vi "Write Sleep TS.vi"(8 "error in (no error)":errorcluster, 10 "Sleep":u64, 11 "CIFCorePlugin in":refnum<class "CIFCorePlugin.lvclass">) -> (0 "error out":errorcluster, 3 "CIFCorePlugin out":refnum<class "CIFCorePlugin.lvclass">)   [LabVIEW 2021, in "CIFCorePlugin.lvclass"]
doc: "Update the timestamp. Time is U64, absolute time in nS in the appropriate clockID configured for the plugin. If a 0 is wired it will automatically get the current time."
uses:
  CIFCorePlugin.lvclass
  CIFCorePlugin.lvclass/CIFCorePlugin.ctl
  CIFUtilities/CIFClocks/Time Conversion/LabVIEW Time to UTC Time.vi
  CIFUtilities/CIFClocks/SubVIs/Add Error.vi
  CIFUtilities/CIFClocks/CIFClocks.lvlib
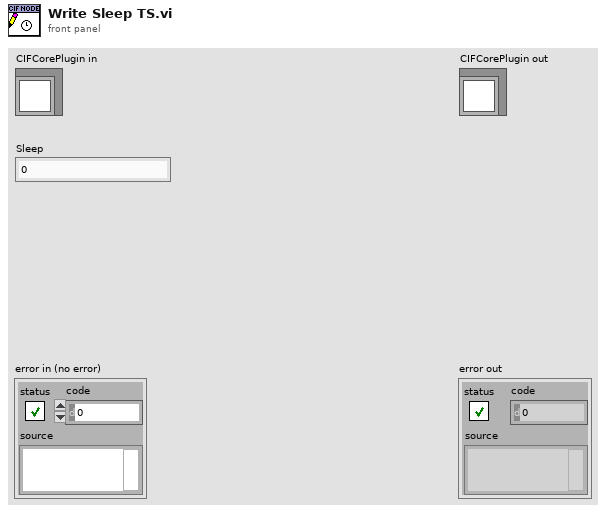
[diagram p1: front panel]
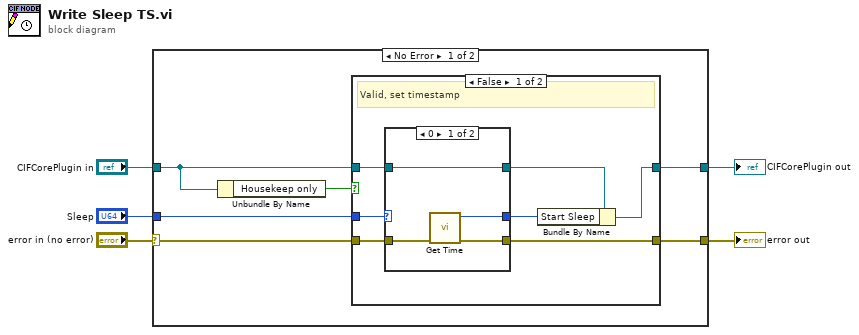
[diagram p0: block diagram]
diagram:
  n1 = case shown="No Error" "error in (no error)" {
    selector: "error in (no error)" -> [w9 w28]
    tunnel: [w8 w28] -> w4
    tunnel: [w11 w29] -> w2
    tunnel: "CIFCorePlugin in" -> [w7 w29]
    tunnel: "Sleep" -> [w10 _]
    frame No Error {
      n2 = Unbundle By Name(w7) -> ("Housekeep only"=w6:bool)
      n3 = case shown="False" w6 {
        tunnel: [w18 w27] -> w11
        tunnel: w10 -> [w17 _]
        tunnel: w9 -> [w16 w26]
        tunnel: [w13 w26] -> w8
        tunnel: w7 -> [w12 w27]
        frame False {
          # "Valid, set timestamp"
          n4 = case shown="0" w17 {
            selector: w17 -> [_ w24]
            tunnel: w16 -> [w21 w23]
            tunnel: w12 -> [w22 w25]
            tunnel: [w22 w25] -> w15
            tunnel: [w20 w24] -> w14
            tunnel: [w19 w23] -> w13
            frame 0 {
              n5 = call "Get Time.vi"("error in (no error)"=w21) -> ("error out"=w19:errorcluster, "Time (ns)"=w20:u64)  [unwired: 8 in, 1 out]
            }
            frame 1, Default {
            }
          }
          n6 = Bundle By Name(cluster=w15, "Start Sleep"=w14) -> (w18:refnum<class "CIFCorePlugin.lvclass">)
        }
        frame True {
          # "Last cycle was housekeeping only, don't set timestamp for benchmark"
        }
      }
    }
    frame Error {
    }
  }
  "error out" <- w4
  "CIFCorePlugin out" <- w2
